vi "VI Properties Editor.vi"() -> ()   [LabVIEW 2020, in "VI Properties Editor.lvlib"]
doc: "Displays a window to add and edit properties and documentation of VIs and their individual controls."
uses:
  VI Properties Editor.lvlib
  Classes/Tree Map/Project Tree Map.lvclass
  Classes/Item/Item.lvclass
  CTLs/Main State Data.ctl
  CTLs/Main Front Panel Controls.ctl
  CTLs/Config.ctl
  <vilib>/Utility/miscctls.llb/LVSelectionTypeDef.ctl
  CTLs/Filter Type.ctl
  CTLs/Filter Column.ctl
  CTLs/Filter Info.ctl
  CTLs/Main References.ctl
  CTLs/Sort Info.ctl
  CTLs/Sort Column.ctl
panel:
  in  "Source Tree":string(tree)
  in  "Help Used":enum32{"Local Help File", "Web-based Help"}(tab)
  in  "Help tag":string
  in  "Help path":string
  in  "Help URL":string
  in  "View Saved Value":bool
  out "VI Type":string
  in  "Edit Icon":bool
  out "Preferred Exec System":string
  out "Priority":string
  out "Suspend when called?":bool
  out "Run when opened?":bool
  out "Auto error handling?":bool
  out "Allow debugging?":bool
  out "Reentrancy":string
  in  "Same as VI name":bool
  in  "Window title":string
  in  "Add Copyright":bool
  out "Inlined?":bool
  in  "Set all VIs":bool
  out "Location":string
  in  "VI description":string
  out "VI Connector Pane":picture
  in  "Controls":string[][](table)
  out "Current Filter":string
  out "Current Counts":string
  out "Current Source":string
  # "Select a VI to view/edit properties:"
  # "Controls"
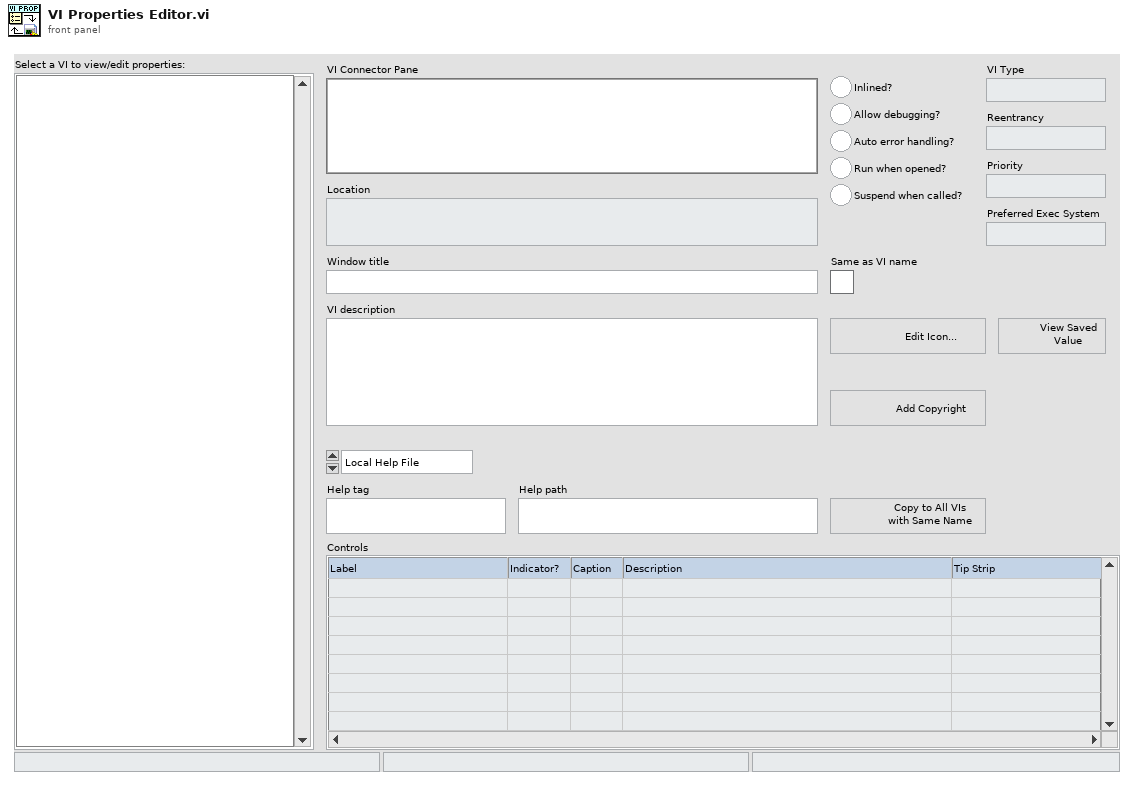
[diagram p1: front panel]
types:
  T1 = typedef "VI Properties Editor.lvlib/Main State Data.ctl" = cluster{"Core":cluster{"Current VI Reference":refnum<vi>, "Close Panel on Exit?":bool}, "FP Refs":T2, "Current Path":path, "New Item Data":refnum<class "Item.lvclass">[], "Saved Item Data":refnum<class "Item.lvclass">[], "FP":T3, "Config Path":path, "Config":T4, "Desc Selection":T8, "Displayed Indices":i32[], "Filter":T5, "Sort":T9, "Tree Map":refnum<class "Project Tree Map.lvclass">, "Last Save Count":u32, "View Saved?":bool, "Selected Item":refnum<class "Item.lvclass">}
  T2 = typedef "VI Properties Editor.lvlib/Main References.ctl" = cluster{"VI Tree":refnum<vi>, "Window Title":refnum<vi>, "Same Title as VI?":refnum<vi>, "VI Desc":refnum<vi>, "Help Path":refnum<vi>, "Help Tag":refnum<vi>, "Help URL":refnum<vi>, "Controls":refnum<vi>, "VI Connector Pane":refnum<vi>, "Path to VI":refnum<vi>, "Inlined?":refnum<vi>, "Allow Debugging?":refnum<vi>, "Auto Error Handling?":refnum<vi>, "Run When Opened?":refnum<vi>, "Suspend When Called?":refnum<vi>, "Reentrancy":refnum<vi>, "Priority":refnum<vi>, "Preferred Exec System":refnum<vi>, "VI Type":refnum<vi>, "Edit Icon":refnum<vi>, "Add Copyright":refnum<vi>, "Set all VIs":refnum<vi>, "Help Used":refnum<vi>}
  T3 = typedef "VI Properties Editor.lvlib/Main Front Panel Controls.ctl" = cluster{"Selected VI Data":i32, "Help Path":string, "Help Tag":string, "Help URL":string, "Help Type":enum16{"Local Help File", "Web-based Help"}, "VI Desc":string, "Controls":string[][], "Window Title":string, "Same Title?":bool, "VI Tree Value":string}
  T4 = typedef "VI Properties Editor.lvlib/Config.ctl" = cluster{"ItemsEdited":u32, "Copyright Path":path, "Copyright Delimiter":string, "Recent Folders":path[], "Recent Files":path[], "Recent Filters":T5[], "Abbreviate Names?":bool, "Format Bold Tags?":bool, "Show ConPane Only?":bool, "Show Top-Level Only?":bool, "Confirm Save?":bool, "Confirm Revert?":bool, "Confirm Save All?":bool, "Confirm Revert All?":bool, "Confirm Exit?":bool, "Flat View?":bool, "Ctls Sort Column":i32, "Ctls Sort Order":i32}
  T5 = typedef "VI Properties Editor.lvlib/Filter Info.ctl" = cluster{"Filter Column":T6, "Filter Type":T7, "Filter Value":string, "New Data?":bool, "Case Sensitive?":bool, "Enabled?":bool}
  T6 = typedef "VI Properties Editor.lvlib/Filter Column.ctl" = enum16{"Name", "Path", "Type", "Window Title", "Description", "Help Path", "Help Tag", "Custom Title?", "Reentrancy", "Inlined?", "Help URL", "Help Type", "Allow Debugging?", "Auto Error Handling?", "Run When Opened?", "Suspend When Called?", "Priority", "Preferred Exec Sytem", "Control Label", "Control Caption", "Control Description", "Control Tip Strip"}
  T7 = typedef "VI Properties Editor.lvlib/Filter Type.ctl" = enum16{"Contains", "Equals", "Starts with", "Ends with", "Is empty", "Does not contain", "Does not equal", "Is not empty"}
  T8 = typedef "LVSelectionTypeDef.ctl" = cluster{"Selection Start":u32, "Selection End":u32}
  T9 = typedef "VI Properties Editor.lvlib/Sort Info.ctl" = cluster{"Sort Column":T10, "Ascending?":bool, "Enabled?":bool}
  T10 = typedef "VI Properties Editor.lvlib/Sort Column.ctl" = enum16{"Name", "Filename", "Path", "Type", "Window Title", "Description", "Help Path", "Help Tag", "Custom Title?", "Reentrancy", "Inlined?", "Help URL", "Help Type", "Allow Debugging?", "Auto Error Handling?", "Run When Opened?", "Suspend When Called?", "Priority", "Preferred Exec Sytem"}
  T11 = enum16{"Text", "Background", "Item Symbol", "Open/Close Symbol", "Hierarchy Lines", "Right Border", "Bottom Border", "Bottom Right Corner", "Unknown Part"}
  T12 = typedef "LVPoint32TypeDef.ctl" = cluster{"Horizontal":i32, "Vertical":i32}
  T13 = cluster{"State(s) at Back":string, "Variant":variant}
  T14 = enum32{"Invalid", "Standard", "Closed", "Hidden", "Minimized", "Maximized"}
  T15 = enum32{"invalid app kind", "Development System", "Run Time System", "Student Edition", "Embedded LabVIEW", "Evaluation", "Custom"}
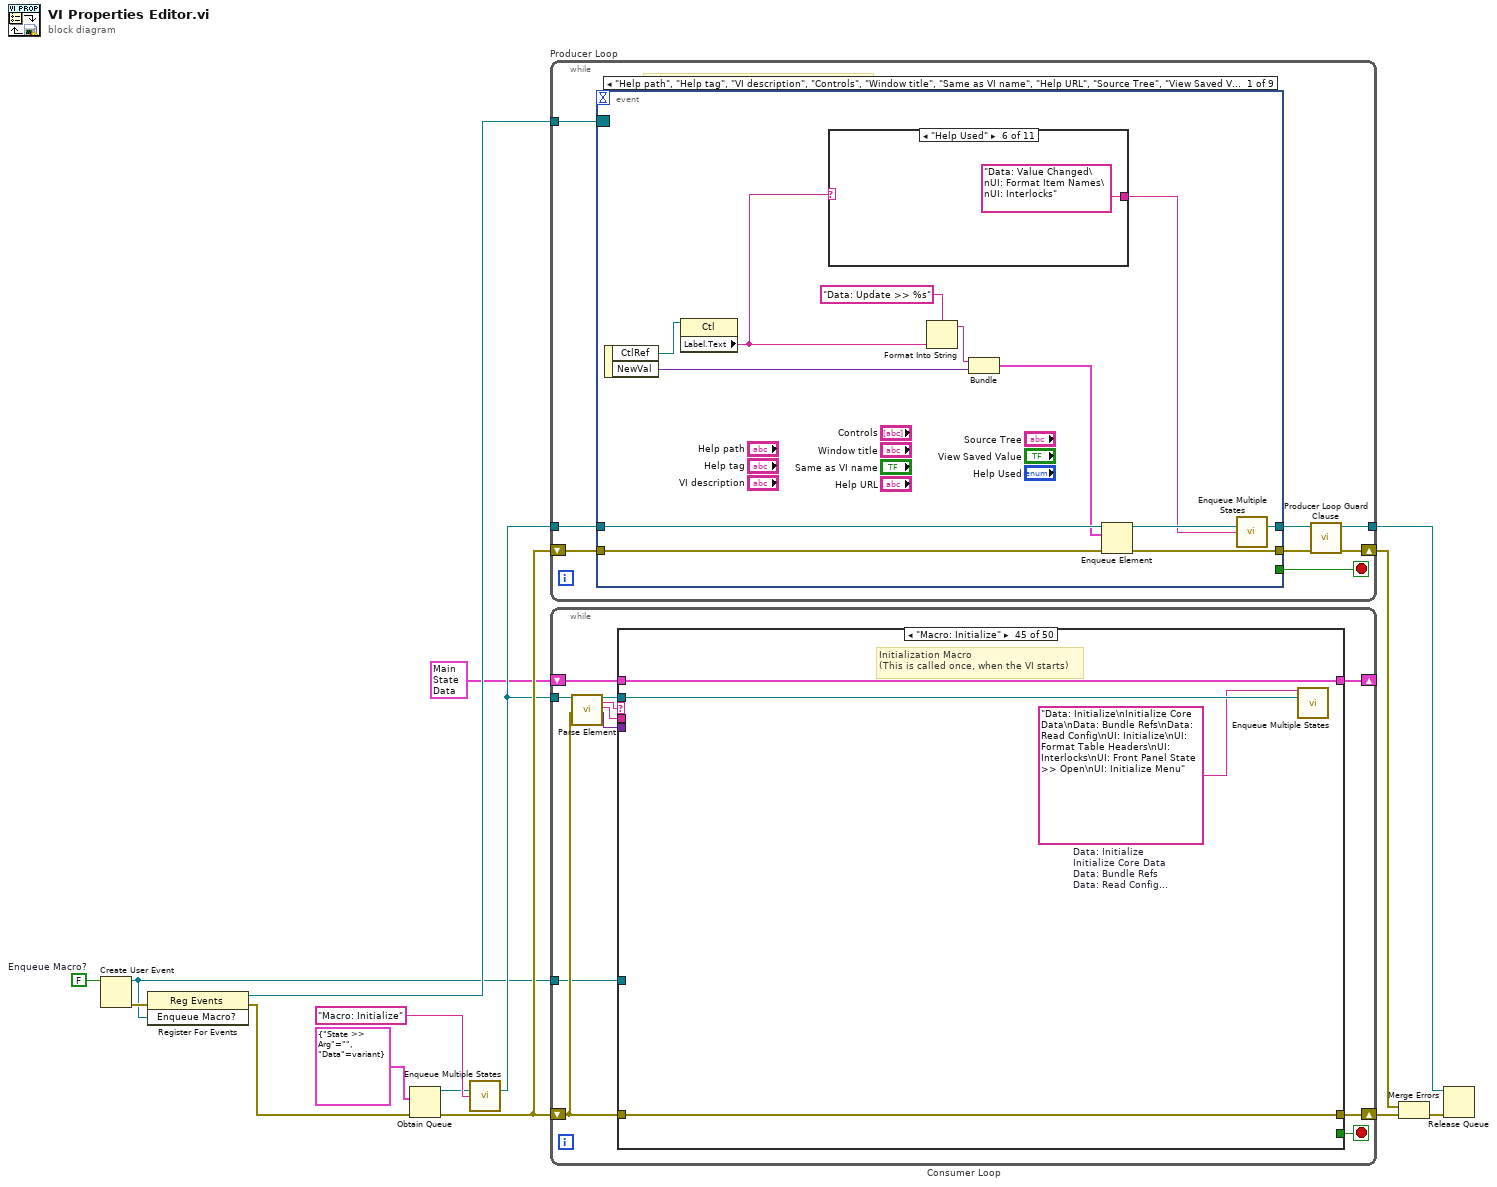
[diagram p0: block diagram]
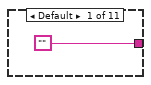
[diagram p2: hidden frame]
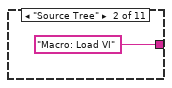
[diagram p3: hidden frame]
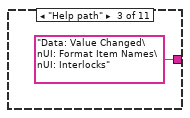
[diagram p4: hidden frame]
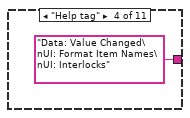
[diagram p5: hidden frame]
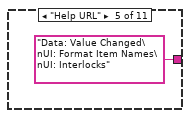
[diagram p6: hidden frame]
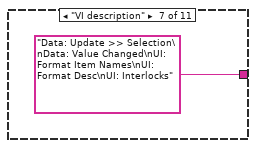
[diagram p7: hidden frame]
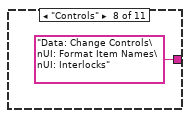
[diagram p8: hidden frame]
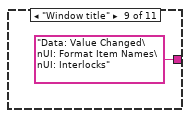
[diagram p9: hidden frame]
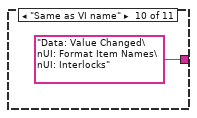
[diagram p10: hidden frame]
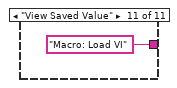
[diagram p11: hidden frame]
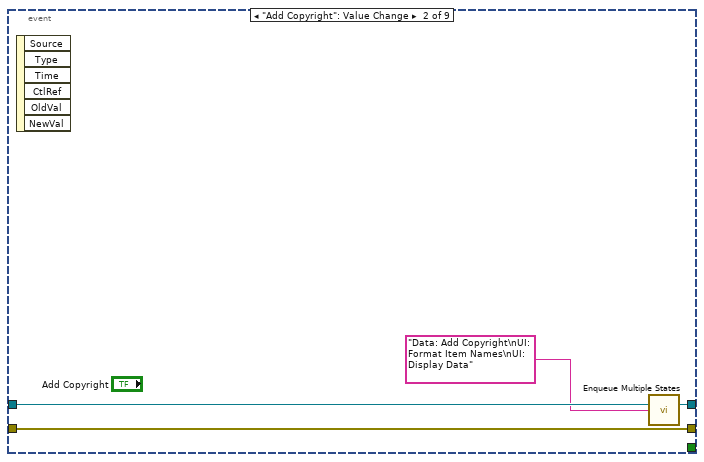
[diagram p12: hidden frame]
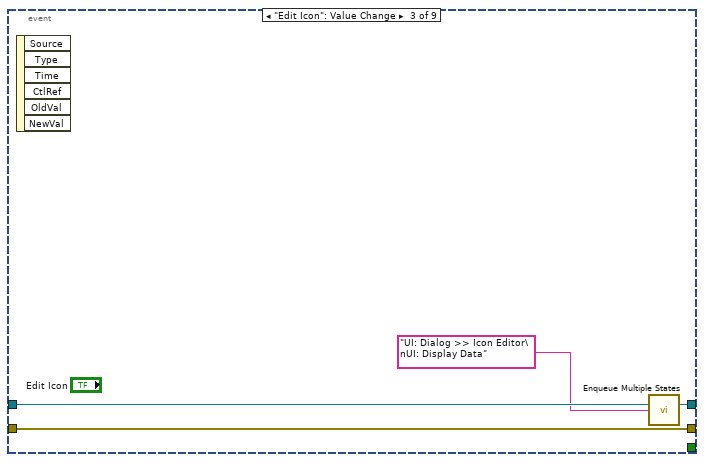
[diagram p13: hidden frame]
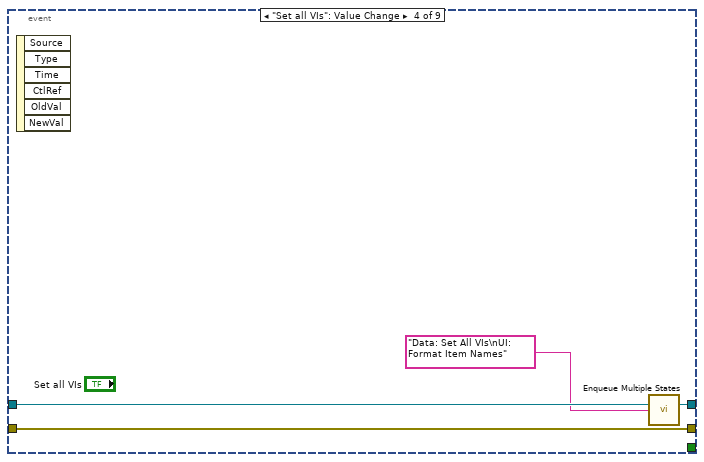
[diagram p14: hidden frame]
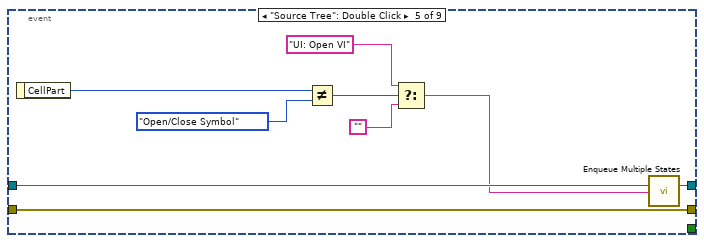
[diagram p15: hidden frame]
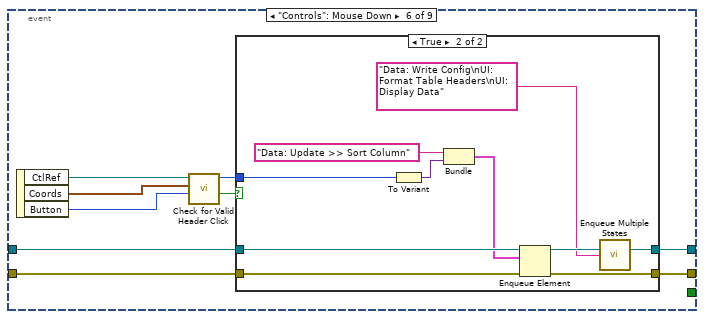
[diagram p16: hidden frame]
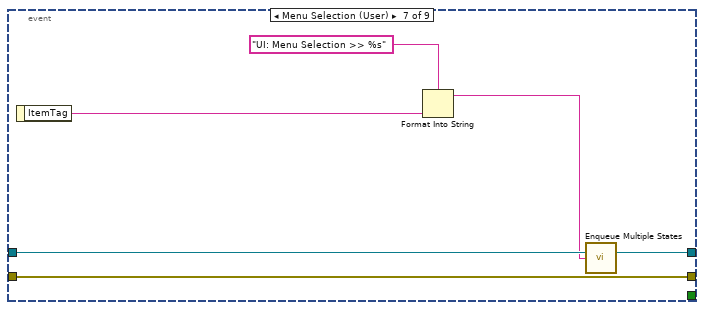
[diagram p18: hidden frame]
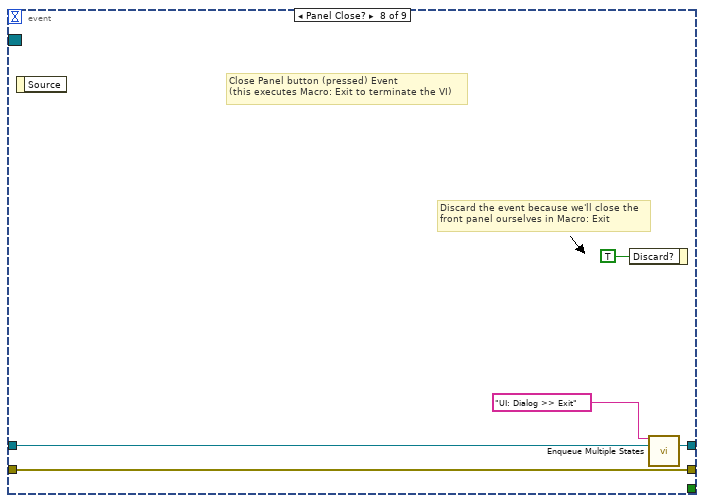
[diagram p19: hidden frame]
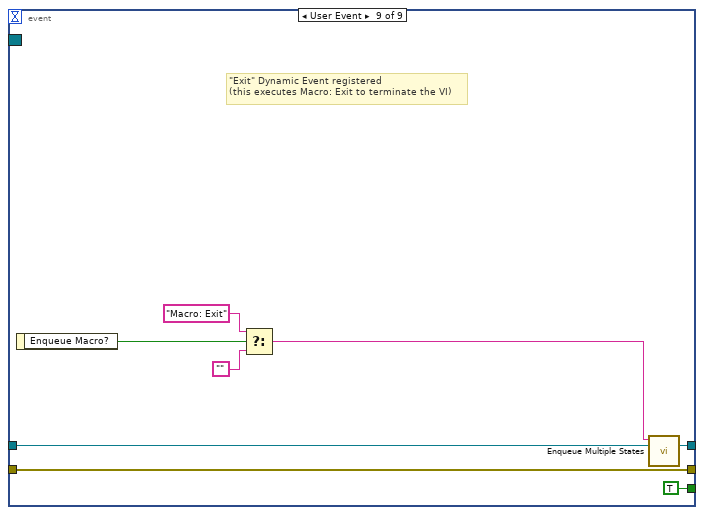
[diagram p20: hidden frame]
diagram:
  w5 = FALSE  # Enqueue Macro?
  n1 = Create User Event(user event datatype=w5) -> (user event=w2:refnum<user-event>, error out=w6:errorcluster)  [unwired: 1 in]
  n2 = register-events(error in=w6, w2) -> (reference out=w3:refnum<event-registration>, error out=w4:errorcluster)  [unwired: 1 in]
  n3 = Obtain Queue(element data type=cluster{"State >> Arg":string, "Data":variant} {"State >> Arg"="", "Data"=variant}, error in (no error)=w4) -> (queue out=w12:refnum<queue>, error out=w15:errorcluster)  [unwired: 3 in, 1 out]
  n4 = call "Enqueue Multiple States.vi"("queue in"=w12, "State(s) at Back"="Macro: Initialize") -> ("queue out"=w11:refnum<queue>)  [unwired: 13 in]
  n5 = while "Producer Loop" {
    shift-right: [w19] -> w9
    shift-left: w15 -> [w23]
    tunnel: w3 -> [w16]
    tunnel: w11 -> [w22]
    tunnel: [w17] -> w7
    stop <- w21 stop-if-true
    # "executes when the state queue is empty"
    n6 = event shown="[0] \"Help path\", \"Help tag\", \"VI description\", \"Controls\", \"Window title\", \"Same as VI name\", \"Help URL\", \"Source Tree\", \"View Saved Value\", \"Help Used\": Value Change" {
      selector: w16 -> [_ _ _ _ _ _ _ _ _]
      dyn-events: _ -> [_ _ _ _ _ _ _ _ _]
      timeout: _ -> [_ _ _ _ _ _ _ _ _]
      tunnel: [w33 w48 w52 w56 w65 w75 w92 w99 w107] -> w20
      tunnel: w23 -> [w34 w48 w52 w56 w65 w76 w92 w99 w107]
      tunnel: w22 -> [w32 w49 w53 w57 w66 w74 w91 w96 w106]
      tunnel: [w35 w50 w54 w58 w67 w73 w90 w95 w105] -> w18
      tunnel: [_ _ _ _ _ _ _ _ TRUE] -> w21
      event "Help path", "Help tag", "VI description", "Controls", "Window title", "Same as VI name", "Help URL", "Source Tree", "View Saved Value", "Help Used": Value Change {
        n7 = event-data() -> ("CtlRef"=w30:refnum<vi>, "NewVal"=w24:variant)  [unwired: 1 in]
        n8 = property on="Property Node" class="Ctl"(reference=w30) -> ("Label.Text"=w26:string)  [unwired: 1 in, 2 out]
        n9 = case shown="\"Help Used\"" w26 {
          tunnel: ["" ("Empty String Constant") "Macro: Load VI" "Data: Value Changed\nUI: Format Item Names\nUI: Interlocks" "Data: Value Changed\nUI: Format Item Names\nUI: Interlocks" "Data: Value Changed\nUI: Format Item Names\nUI: Interlocks" "Data: Value Changed\nUI: Format Item Names\nUI: Interlocks" "Data: Update >> Selection\nData: Value Changed\nUI: Format Item Names\nUI: Format Desc\nUI: Interlocks" "Data: Change Controls\nUI: Format Item Names\nUI: Interlocks" "Data: Value Changed\nUI: Format Item Names\nUI: Interlocks" "Data: Value Changed\nUI: Format Item Names\nUI: Interlocks" "Macro: Load VI"] -> w25
          frame Default {
          }
          frame "Source Tree" {
          }
          frame "Help path" {
          }
          frame "Help tag" {
          }
          frame "Help URL" {
          }
          frame "Help Used" {
          }
          frame "VI description" {
          }
          frame "Controls" {
          }
          frame "Window title" {
          }
          frame "Same as VI name" {
          }
          frame "View Saved Value" {
          }
        }
        n10 = Format Into String(format string="Data: Update >> %s", w26) -> (resulting string=w28:string)  [unwired: 2 in, 1 out]
        n11 = Bundle(w28, "NewVal"=w24) -> (w27:cluster{string, "NewVal":variant})  [unwired: 1 in]
        n12 = Enqueue Element(queue=w32, element=w27, error in (no error)=w34) -> (queue out=w31:refnum<queue>, error out=w33:errorcluster)  [unwired: 1 in, 1 out]
        n13 = call "Enqueue Multiple States.vi"("queue in"=w31, "State(s) at Back"=w25) -> ("queue out"=w35:refnum<queue>)  [unwired: 13 in]
      }
      event "Add Copyright": Value Change {
        n14 = event-data() -> ()  [unwired: 1 in, 6 out]
        n15 = call "Enqueue Multiple States.vi"("queue in"=w49, "State(s) at Back"="Data: Add Copyright\nUI: Format Item Names\nUI: Display Data") -> ("queue out"=w50:refnum<queue>)  [unwired: 13 in]
      }
      event "Edit Icon": Value Change {
        n16 = event-data() -> ()  [unwired: 1 in, 6 out]
        n17 = call "Enqueue Multiple States.vi"("queue in"=w53, "State(s) at Back"="UI: Dialog >> Icon Editor\nUI: Display Data") -> ("queue out"=w54:refnum<queue>)  [unwired: 13 in]
      }
      event "Set all VIs": Value Change {
        n18 = event-data() -> ()  [unwired: 1 in, 6 out]
        n19 = call "Enqueue Multiple States.vi"("queue in"=w57, "State(s) at Back"="Data: Set All VIs\nUI: Format Item Names") -> ("queue out"=w58:refnum<queue>)  [unwired: 13 in]
      }
      event "Source Tree": Double Click {
        n20 = event-data() -> ("CellPart"=w64:T11)  [unwired: 1 in]
        n21 = Not Equal?(x=w64, y=T11."Open/Close Symbol") -> (x != y?=w62:bool)
        n22 = Select(t="UI: Open VI" ("State(s) at Back"), s=w62, f="" ("Empty String Constant")) -> (s? t:f=w59:string)
        n23 = call "Enqueue Multiple States.vi"("queue in"=w66, "State(s) at Back"=w59) -> ("queue out"=w67:refnum<queue>)  [unwired: 13 in]
      }
      event "Controls": Mouse Down {
        n24 = event-data() -> ("CtlRef"=w72:refnum<vi>, "Coords"=w71:T12, "Button"=w70:u16)  [unwired: 1 in]
        n25 = call "Check for Valid Header Click.vi"("Button"=w70, "Coords"=w71, "Table Ref"=w72) -> ("Valid Click?"=w69:bool, "Column"=w68:i32)  [unwired: 7 in]
        n26 = case shown="True" w69 {
          tunnel: w76 -> [w77 w88]
          tunnel: [w77 w87] -> w75
          tunnel: w74 -> [w78 w85]
          tunnel: [w78 w84] -> w73
          tunnel: w68 -> [_ w81]
          frame False {
          }
          frame True {
            n27 = To Variant(anything=w81) -> (Variant=w83:variant)
            n28 = Bundle("State(s) at Back"="Data: Update >> Sort Column", "Variant"=w83) -> (w80:T13)  [unwired: 1 in]
            n29 = Enqueue Element(queue=w85, element=w80, error in (no error)=w88) -> (queue out=w86:refnum<queue>, error out=w87:errorcluster)  [unwired: 1 in, 1 out]
            n30 = call "Enqueue Multiple States.vi"("queue in"=w86, "State(s) at Back"="Data: Write Config\nUI: Format Table Headers\nUI: Display Data") -> ("queue out"=w84:refnum<queue>)  [unwired: 13 in]
          }
        }
      }
      event Menu Selection (User) {
        n31 = event-data() -> ("ItemTag"=w93:string)  [unwired: 1 in]
        n32 = Format Into String(format string="UI: Menu Selection >> %s", w93) -> (resulting string=w89:string)  [unwired: 2 in, 1 out]
        n33 = call "Enqueue Multiple States.vi"("queue in"=w91, "State(s) at Back"=w89) -> ("queue out"=w90:refnum<queue>)  [unwired: 13 in]
      }
      event Panel Close? {
        # "Discard the event because we'll close the front panel ourselves in Macro: Exit"
        # "Close Panel button (pressed) Event\n(this executes Macro: Exit to terminate the VI)"
        n34 = event-data() -> ()  [unwired: 1 in, 1 out]
        n35 = event-data ("Event Filter Node")("Discard?"=TRUE) -> ()  [unwired: 1 in, 1 out]
        n36 = call "Enqueue Multiple States.vi"("State(s) at Front"="UI: Dialog >> Exit", "queue in"=w96) -> ("queue out"=w95:refnum<queue>)  [unwired: 13 in]
      }
      event User Event {
        # "\"Exit\" Dynamic Event registered\n(this executes Macro: Exit to terminate the VI)"
        n37 = event-data() -> ("Enqueue Macro?"=w103:bool)  [unwired: 1 in]
        n38 = Select(t="Macro: Exit", s=w103, f="" ("Empty String Constant")) -> (s? t:f=w100:string)
        n39 = call "Enqueue Multiple States.vi"("State(s) at Front"=w100, "queue in"=w106) -> ("queue out"=w105:refnum<queue>)  [unwired: 13 in]
      }
    }
    n40 = call "Producer Loop Guard Clause.vi"("error in (no error)"=w20, "queue in"=w18) -> ("error out"=w19:errorcluster, "queue out"=w17:refnum<queue>)  [unwired: 8 in]
  }
  n41 = while "Consumer Loop" {
    shift-right: [w115] -> _
    shift-left: T1 {"Core"={"Current VI Reference"=refnum, "Close Panel on Exit?"=FALSE}, "FP Refs"={"VI Tree"=refnum, "Window Title"=refnum, "Same Title as VI?"=refnum, "VI Desc"=refnum, "Help Path"=refnum, "Help Tag"=refnum, "Help URL"=refnum, "Controls"=refnum, "VI Connector Pane"=refnum, "Path to VI"=refnum, "Inlined?"=refnum, "Allow Debugging?"=refnum, "Auto Error Handling?"=refnum, "Run When Opened?"=refnum, "Suspend When Called?"=refnum, "Reentrancy"=refnum, "Priority"=refnum, "Preferred Exec System"=refnum, "VI Type"=refnum, "Edit Icon"=refnum, "Add Copyright"=refnum, "Set all VIs"=refnum, "Help Used"=refnum}, "Current Path"=path "", "New Item Data"=[], "Saved Item Data"=[], "FP"={"Selected VI Data"=0, "Help Path"="", "Help Tag"="", "Help URL"="", "Help Type"=enum."Local Help File", "VI Desc"="", "Controls"=[], "Window Title"="", "Same Title?"=FALSE, "VI Tree Value"=""}, "Config Path"=path "", "Config"={"ItemsEdited"=0, "Copyright Path"=path "", "Copyright Delimiter"="", "Recent Folders"=[], "Recent Files"=[], "Recent Filters"=[], "Abbreviate Names?"=FALSE, "Format Bold Tags?"=FALSE, "Show ConPane Only?"=FALSE, "Show Top-Level Only?"=FALSE, "Confirm Save?"=FALSE, "Confirm Revert?"=FALSE, "Confirm Save All?"=FALSE, "Confirm Revert All?"=FALSE, "Confirm Exit?"=FALSE, "Flat View?"=FALSE, "Ctls Sort Column"=0, "Ctls Sort Order"=0}, "Desc Selection"={"Selection Start"=0, "Selection End"=0}, "Displayed Indices"=[], "Filter"={"Filter Column"=enum."Name", "Filter Type"=enum."Contains", "Filter Value"="", "New Data?"=FALSE, "Case Sensitive?"=FALSE, "Enabled?"=FALSE}, "Sort"={"Sort Column"=enum."Name", "Ascending?"=FALSE, "Enabled?"=FALSE}, "Tree Map"=refnum, "Last Save Count"=0, "View Saved?"=FALSE, "Selected Item"=refnum} ("VI Properties Editor State Data") -> [w114]
    shift-right: [w118] -> w10
    shift-left: w15 -> [w117]
    tunnel: w11 -> [w113]
    tunnel: w2 -> [w108]
    stop <- w116 stop-if-true
    n42 = call "Parse Element.vi"("queue in"=w113, "error in (no error)"=w117) -> ("queue out"=w112:refnum<queue>, "State"=w111:string, "Arg"=w110:string, "Data"=w109:variant)  [unwired: 14 in]
    n43 = case shown="\"Macro: Initialize\"" w111 {
      selector: w111 -> [_ w121 _ _ _ _ _ _ _ _ _ _ _ _ _ _ _ _ _ _ _ _ _ _ _ _ _ _ _ _ _ _ _ _ _ _ _ _ _ _ _ _ _ _ _ _ _ _ _ _]
      tunnel: w112 -> [_ _ _ _ _ _ _ _ _ w216 _ w223 _ _ _ _ _ _ _ _ _ _ _ _ _ _ _ w399 _ _ _ _ w502 _ _ w544 _ _ _ _ _ _ _ _ w662 w666 w671 w684 w691 w703]
      tunnel: w110 -> [_ _ _ w146 _ _ _ _ w201 _ _ w224 w232 _ _ _ _ _ _ _ _ w353 _ _ _ _ _ w394 w401 w409 w481 _ w497 _ _ w531 _ _ _ _ _ w612 w651 _ _ _ w670 w682 w689 _]
      tunnel: w114 -> [w119 w123 w140 w150 w153 w155 w169 w199 w203 w212 w219 w227 w235 w262 w277 w286 w294 w300 w311 w332 w340 w356 w370 w374 w377 w388 w390 w400 w402 w411 w486 w494 w499 w523 w529 w542 w560 w573 w584 w595 w603 w610 w649 w659 w663 w667 w672 w681 w688 w707]
      tunnel: [w120 w128 w145 errorcluster {"status"=FALSE, "code"=0, "source"=""} ("error out") w154 w156 w162 w197 w204 w214 w220 w228 w238 w259 w278 w287 w295 w298 w308 w333 w341 w362 w372 w375 w378 w380 w392 w397 w403 w412 w482 w491 w500 w518 w527 w533 w561 w574 w580 w591 w602 w615 w653 w660 w664 w668 w673 w680 w687 w696] -> w118
      tunnel: w117 -> [w120 w127 w145 w149 w154 w156 w161 w197 w205 w215 w221 w229 w237 w260 w278 w287 w295 w299 w309 w333 w341 w358 w373 w375 w378 w383 w393 w398 w404 w413 w483 w492 w501 w514 w528 w535 w562 w575 w581 w592 w607 w614 w652 w660 w664 w668 w673 w680 w687 w708]
      tunnel: [_ _ _ _ TRUE _ _ _ _ _ _ _ _ _ _ _ _ _ _ _ _ _ _ _ _ _ _ _ _ _ _ _ _ _ _ _ _ _ _ _ _ _ _ _ _ _ _ _ _ _] -> w116
      tunnel: [w119 w123 w144 w150 w153 w155 w168 w198 w202 w213 w219 w227 w234 w261 w276 w285 w293 w297 w312 w334 w342 w361 w370 w374 w377 w388 w390 w400 w402 w411 w486 w494 w498 w523 w529 w541 w560 w573 w583 w594 w603 w611 w650 w659 w663 w667 w672 w681 w688 w707] -> w115
      tunnel: w109 -> [_ _ _ w147 _ _ _ _ w200 _ _ _ _ _ _ _ _ _ _ _ _ _ _ _ _ _ _ _ _ _ _ _ _ _ _ _ _ _ _ _ _ _ _ _ _ _ _ _ _ _]
      tunnel: w108 -> [_ _ _ _ _ _ _ _ _ _ _ _ _ _ _ _ _ _ _ _ _ _ _ _ _ _ _ _ _ _ _ _ _ _ _ _ _ _ _ _ _ _ _ _ _ _ _ _ _ w699]
      frame "---------- Core ----------" {
        # "Do not put any code in this frame.\n(it is a separator no-op)"
      }
      frame Default {
        w125 = 42 items=["No error", "Argument error", "Memory is full", "Out of zone", "End of file", "File already open", "Generic file I/O error", "File not found", "File permission error", "Disk is full", "Duplicate path", "Too many files open", "System feature not enabled", "Resource file not found", "Cannot add resource", "Resource not found", "Image not found", "Image memory error", "Pen does not exist", "Config type invalid", "Config token not found", "Config parse error", "Config memory error", "Bad external code format", "Bad external code offset", "External code not present", "Null window", "Destroy window error", "Null menu", "Print aborted", "Bad print record", "Print driver error", "Windows error during printing", "Memory error during printing", "Print dialog error", "Generic print error", "Invalid device refnum", "Device not found", "Device parameter error", "Device unit error", "Cannot open device", "Device call aborted", "Generic error", "Cancelled by user", "Object ID too low", "Object ID too high", "Object not in heap", "Unknown heap", "Unknown object (invalid DefProc)", "Unknown object (DefProc not in table)", "Message out of range", "Invalid (null) method", "Unknown message", "Manager call not supported", "Bad address", "Network operation in progress", "Network operation timed out", "Connection is busy", "Network attribute not supported", "Network error", "Address in use", "System out of memory", "Connection aborted", "Connection refused", "Not connected", "Already connected", "Connection closed", "Initialization error (interapplication manager)", "Bad occurrence", "Wait on unbound occurrence handler", "Occurrence queue overflow", "Datalog type conflict", "Unused", "Unrecognized type (interapplication manager)", "Memory corrupt", "Failed to make temporary DLL", "Old CIN version", "Drag socket not found", "Failed to load drop-object", "Failed to register OLE object", "Failed to release OLE object", "Format specifier type mismatch", "Unknown format specifier", "Too few format specifiers", "Too many format specifiers", "Scan failed", "Newer CIN version", "Error converting to variant", "Runtime menu error", "Password tampered", "Variant attribute not found", "Incompatible variant data type", "Event data is not available", "Event Store is not present", "Occurrence is not found", "Event Queue is not created", "Event info is not available", "Refnum passed is NULL", "Error retrieving Class GUID", "Error retrieving CoClass GUID", "Error retrieving TypeLib GUID.", "Bad built application magic bytes.", "Specific driver is different from the specific driver associated with the Logical Name.", "There is no session opened to the class driver.", "Max Error", "MAX - Error with config objects", "MAX - Error loading configuration", "MAX - Group not supported"]
        # "Current State"
        # "Do not delete, rename, or modify this frame.\n(this is used to capture unhandled states and typos)"
        # "Handle mistyped state name (developer tool)"
        n44 = Format Into String(format string="Software Exception: Unhandled State \"%s\"." ("message"), error in=w127, w121) -> (resulting string=w124:string, error out=w129:errorcluster)  [unwired: 1 in]
        n45 = call <vilib>:"Error Cluster From Error Code.vi"("show call chain? (False)"=TRUE, "error in (no error)"=w129, "error message (\"\")"=w124, "error code (0)"=w125) -> ("error out"=w128:errorcluster)  [unwired: 5 in]
      }
      frame "Initialize Core Data" {
        # "Want the VI to close when ran from the Tools menu"
        # "originally closed?"
        # "exe?"
        # "If panel starts closed or is an EXE, then close it when we exit"
        n46 = property on="Property Node" class="VI"() -> ("FP.State"=w137:T14)  [unwired: 2 in, 2 out]
        n47 = property on="Property Node" class="App"() -> ("App.Kind"=w143:T15)  [unwired: 2 in, 2 out]
        n48 = Current VI's Path() -> (path=w134:path)
        n49 = control-ref of="Current VI Reference"() -> (w138:refnum<vi>)
        n50 = Strip Path(path=w134) -> (stripped path=w133:path)  [unwired: 1 out]
        n51 = Equal?(x=w137, y=T14."Closed" ("Front Panel Window:State")) -> (x = y?=w135:bool)
        n52 = Equal?(x=w143, y=T15."Run Time System" ("Application:Kind")) -> (x = y?=w141:bool)
        n53 = Strip Path(path=w133) -> (name=w132:string)  [unwired: 1 out]
        n54 = Equal?(x=w132, y="Redhawk" ("name")) -> (x = y?=w130:bool)
        n55 = Compound Arithmetic op=OR(w135, w141, w130) -> (w139:bool)
        n56 = Bundle By Name(cluster=w140, "Core.Current VI Reference"=w138, "Core.Close Panel on Exit?"=w139) -> (w144:T1)
      }
      frame "Error Handler" {
        # "Unhandled Error -- Display it"
        # "Handle any errors here.\nYou can also output any states to clean-up after errors occur"
        # "Clear error"
        n57 = call "Build Error Message.vi"("error in (no error)"=w149, "Data"=w147, "Arg"=w146) -> ("error out"=w148:errorcluster)  [unwired: 8 in]
        n58 = call <vilib>:"General Error Handler.vi"("error in (no error)"=w148) -> ()  [unwired: 10 in, 5 out]
      }
      frame "Exit" {
        # "Do not put any code in this frame.\n(No errors that occur here will be handled.)"
      }
      frame "---------- Data ----------" {
        # "Do not put any code in this frame.\n(It is a separator no-op. You can make a copy of this frame to create a new Data frame)"
      }
      frame "Data: Initialize" {
        # "Initialize the shift-register data, here."
        n59 = call "Config Path--constant.vi"() -> ("Config Path"=w158:path)  [unwired: 11 in]
        n60 = Strip Path(path=w158) -> (stripped path=w166:path)  [unwired: 1 out]
        n61 = call <vilib>:"Check if File or Folder Exists.vi"("error in (no error)"=w161, "path"=w166) -> ("error out"=w165:errorcluster, "file or folder exists?"=w163:bool, "dup path"=w164:path)  [unwired: 7 in]
        n62 = case shown="True" w163 {
          tunnel: [w172 w173] -> w162
          tunnel: w165 -> [w171 w173]
          tunnel: w164 -> [w170 _]
          frame False {
            n63 = Create Folder(path (use dialog)=w170, error in=w171) -> (error out=w172:errorcluster)  [unwired: 1 in, 2 out]
          }
          frame True {
          }
        }
        n64 = Bundle By Name(cluster=w169, "FP.Selected VI Data"=-1 ("FP.VI Selected"), "Sort.Sort Column"=Sort_Column."Name", "Sort.Ascending?"=TRUE ("Ascending?"), "Sort.Enabled?"=FALSE ("Ascending?"), "Config Path"=w158) -> (w168:T1)
      }
      frame "Data: Bundle Refs" {
        n65 = control-ref of="Source Tree"() -> (w196:refnum<vi>)
        n66 = control-ref of="Help Used"() -> (w178:refnum<vi>)
        n67 = control-ref of="Same as VI name"() -> (w194:refnum<vi>)
        n68 = control-ref of="Inlined?"() -> (w186:refnum<vi>)
        n69 = control-ref of="Allow debugging?"() -> (w185:refnum<vi>)
        n70 = control-ref of="Auto error handling?"() -> (w184:refnum<vi>)
        n71 = control-ref of="Run when opened?"() -> (w183:refnum<vi>)
        n72 = control-ref of="Suspend when called?"() -> (w182:refnum<vi>)
        n73 = control-ref of="Edit Icon"() -> (w177:refnum<vi>)
        n74 = control-ref of="Add Copyright"() -> (w176:refnum<vi>)
        n75 = control-ref of="Set all VIs"() -> (w175:refnum<vi>)
        n76 = control-ref of="VI Connector Pane"() -> (w189:refnum<vi>)
        n77 = control-ref of="Window title"() -> (w195:refnum<vi>)
        n78 = control-ref of="VI description"() -> (w193:refnum<vi>)
        n79 = control-ref of="Help path"() -> (w192:refnum<vi>)
        n80 = control-ref of="Help tag"() -> (w191:refnum<vi>)
        n81 = control-ref of="Help URL"() -> (w187:refnum<vi>)
        n82 = control-ref of="Location"() -> (w188:refnum<vi>)
        n83 = control-ref of="Reentrancy"() -> (w181:refnum<vi>)
        n84 = control-ref of="Priority"() -> (w180:refnum<vi>)
        n85 = control-ref of="Preferred Exec System"() -> (w179:refnum<vi>)
        n86 = control-ref of="VI Type"() -> (w174:refnum<vi>)
        n87 = control-ref of="Controls"() -> (w190:refnum<vi>)
        n88 = Bundle By Name(cluster=w199, "FP Refs.VI Tree"=w196, "FP Refs.Window Title"=w195, "FP Refs.Same Title as VI?"=w194, "FP Refs.VI Desc"=w193, "FP Refs.Help Path"=w192, "FP Refs.Help Tag"=w191, "FP Refs.Help URL"=w187, "FP Refs.Controls"=w190, "FP Refs.VI Connector Pane"=w189, "FP Refs.Path to VI"=w188, "FP Refs.Inlined?"=w186, "FP Refs.Allow Debugging?"=w185, "FP Refs.Auto Error Handling?"=w184, "FP Refs.Run When Opened?"=w183, "FP Refs.Suspend When Called?"=w182, "FP Refs.Reentrancy"=w181, "FP Refs.Priority"=w180, "FP Refs.Preferred Exec System"=w179, "FP Refs.VI Type"=w174, "FP Refs.Help Used"=w178, "FP Refs.Edit Icon"=w177, "FP Refs.Add Copyright"=w176, "FP Refs.Set all VIs"=w175) -> (w198:T1)
      }
      frame "Data: Update" {
        n89 = call "Update State Data.vi"("error in (no error)"=w205, "Data"=w200, "Argument"=w201, "State Data"=w203) -> ("error out"=w204:errorcluster, "State Data out"=w202:T1)  [unwired: 6 in]
      }
      frame "Data: Read Config" {
        n90 = Unbundle By Name(w212) -> ("Config Path"=w211:path)
        n91 = call "Read Config.vi"("error in (no error)"=w215, "Path"=w211) -> ("error out"=w214:errorcluster, "Config"=w210:T4, "File Created?"=w209:bool)  [unwired: 7 in]
        n92 = Bundle By Name(cluster=w212, "Config"=w210) -> (w213:T1)
        n93 = Select(t="Data: Write Config", s=w209, f="" ("Empty String Constant")) -> (s? t:f=w206:string)
        n94 = call "Enqueue Multiple States.vi"("queue in"=w216, "State(s) at Back"=w206) -> ()  [unwired: 13 in, 1 out]
      }
      frame "Data: Write Config" {
        n95 = Unbundle By Name(w219) -> ("Config Path"=w217:path, "Config"=w218:T4)
        n96 = call "Write Config.vi"("error in (no error)"=w221, "Config"=w218, "Path"=w217) -> ("error out"=w220:errorcluster)  [unwired: 8 in]
      }
      frame "Data: Check Source" {
        n97 = Unbundle By Name(w227) -> ("Config"=w226:T4, "Current Path"=w225:path)
        n98 = call "Check Data Source.vi"("error in (no error)"=w229, "Argument"=w224, "Current Path"=w225, "Config"=w226) -> ("error out"=w228:errorcluster, "States"=w222:string)  [unwired: 6 in]
        n99 = call "Enqueue Multiple States.vi"("queue in"=w223, "State(s) at Back"=w222) -> ()  [unwired: 13 in, 1 out]
      }
      frame "Data: Load VIs" {
        n100 = Unbundle By Name(w235) -> ("Core.Current VI Reference"=w230:refnum<vi>, "Current Path"=w236:path)
        n101 = Equal?(x=w232, y="Reload") -> (x = y?=w231:bool)
        n102 = in-place "In Place Element Structure" {
          in-place-border: [w249] -> w238
          in-place-border: w237 -> [w248]
          in-place-border: w236 -> [w242]
          in-place-border: w231 -> [w244]
          in-place-border: w230 -> [w243]
          n103 = in-place-cluster #1(w235) -> ("New Item Data"=w247:refnum<class "Item.lvclass">[], "Saved Item Data"=w240:refnum<class "Item.lvclass">[])
          n104 = call "Get All Items.vi"("Calling VI Ref"=w243, "error in (no error)"=w248, "Path"=w242) -> ("error out"=w249:errorcluster, "Cancelled?"=w241:bool, "Item Data"=w246:refnum<class "Item.lvclass">[])  [unwired: 6 in]
          n105 = case shown="False" w241 {
            tunnel: w247 -> [w256 w258]
            tunnel: w246 -> [w250 _]
            tunnel: [w255 w258] -> w245
            tunnel: w244 -> [w254 _]
            tunnel: w242 -> [w253 _]
            tunnel: w240 -> [_ w257]
            tunnel: [w250 w257] -> w239
            frame False {
              n106 = Array Size(array=w250) -> (size(s)=w252:i32)
              n107 = Select(t=w256, s=w254, f=w250) -> (s? t:f=w255:refnum<class "Item.lvclass">[])
              n108 = call "Format Current Source String.vi"("Item Count"=w252, "Current Path"=w253) -> ("Current Source String"=→"Current Source":string)  [unwired: 9 in]
            }
            frame True {
            }
          }
          n109 = in-place-cluster #1("New Item Data"=w245, "Saved Item Data"=w239) -> (w234:T1)
        }
      }
      frame "Data: Filter/Sort VIs" {
        n110 = in-place "In Place Element Structure" {
          in-place-border: w260 -> [w269]
          in-place-border: [w268] -> w259
          n111 = in-place-cluster #2(w262) -> ("Sort"=w273:T9, "Filter"=w274:T5, "Saved Item Data"=w265:refnum<class "Item.lvclass">[], "New Item Data"=w266:refnum<class "Item.lvclass">[])  [unwired: 1 out]
          n112 = call "Filter and Sort Items.vi"("Sort Info"=w273, "Filter Info"=w274, "error in (no error)"=w269, "New Item Data"=w266, "Saved Item Data"=w265) -> ("error out"=w268:errorcluster, "Displayed Indices"=w263:i32[], "New Item Data out"=w267:refnum<class "Item.lvclass">[], "Saved Item Data out"=w264:refnum<class "Item.lvclass">[])  [unwired: 3 in]
          n113 = call "Convert Filter to Display String.vi"("Filter Info"=w274) -> ("String"=w270:string)  [unwired: 10 in]
          n114 = Concatenate Strings("Current filter:  " ("string"), w270) -> (→"Current Filter":string)
          n115 = in-place-cluster #2("Sort"=w273, "Filter"=w274, "Saved Item Data"=w264, "New Item Data"=w267, "Displayed Indices"=w263) -> (w261:T1)
        }
      }
      frame "Data: Value Changed" {
        n116 = Unbundle By Name(w277) -> ("FP"=w275:T3)
        n117 = in-place "In Place Element Structure" {
          in-place-border: w275 -> [w280]
          n118 = in-place-cluster #3(w277) -> ("New Item Data"=w279:refnum<class "Item.lvclass">[])
          n119 = call "Set VI Properties.vi"("Front Panel Controls"=w280, "Item Data"=w279) -> ("Item Data out"=w281:refnum<class "Item.lvclass">[])  [unwired: 9 in]
          n120 = in-place-cluster #3("New Item Data"=w281) -> (w276:T1)
        }
      }
      frame "Data: Revert Current" {
        n121 = Unbundle By Name(w286) -> ("FP.Selected VI Data"=w282:i32, "Saved Item Data"=w284:refnum<class "Item.lvclass">[])
        n122 = Index Array(array=w284, index=w282) -> (element=w283:refnum<class "Item.lvclass">)
        n123 = in-place "In Place Element Structure" {
          in-place-border: w283 -> [w290]
          in-place-border: w282 -> [w289]
          n124 = in-place-cluster #4(w286) -> ("New Item Data"=w291:refnum<class "Item.lvclass">[])
          n125 = Replace Array Subset(array=w291, new element=w290, index=w289) -> (w288:refnum<class "Item.lvclass">[])
          n126 = in-place-cluster #4("New Item Data"=w288) -> (w285:T1)
        }
      }
      frame "Data: Revert All" {
        n127 = Unbundle By Name(w294) -> ("Saved Item Data"=w292:refnum<class "Item.lvclass">[])
        n128 = in-place "In Place Element Structure" {
          in-place-border: w292 -> [w296]
          n129 = in-place-cluster #5(w294) -> ()  [unwired: 1 out]
          n130 = in-place-cluster #5("New Item Data"=w296) -> (w293:T1)
        }
      }
      frame "Data: Save All" {
        n131 = in-place "In Place Element Structure" {
          in-place-border: w299 -> [w307]
          in-place-border: [w306] -> w298
          n132 = in-place-cluster #6(w300) -> ("New Item Data"=w303:refnum<class "Item.lvclass">[], "Saved Item Data"=w302:refnum<class "Item.lvclass">[])  [unwired: 1 out]
          n133 = call "Save All VI Data.vi"("error in (no error)"=w307, "Saved Item Data"=w302, "New Item Data"=w303) -> ("error out"=w306:errorcluster, "Items Saved"=w301:u32, "Saved Item Data out"=w304:refnum<class "Item.lvclass">[], "New Item Data out"=w305:refnum<class "Item.lvclass">[])  [unwired: 5 in]
          n134 = in-place-cluster #6("Last Save Count"=w301, "New Item Data"=w305, "Saved Item Data"=w304) -> (w297:T1)
        }
      }
      frame "Data: Save Current" {
        n135 = Unbundle By Name(w311) -> ("FP.Selected VI Data"=w310:i32)
        n136 = in-place "In Place Element Structure" {
          in-place-border: w310 -> [w318]
          in-place-border: w309 -> [w315]
          in-place-border: [w314] -> w308
          n137 = in-place-cluster #7(w311) -> ("New Item Data"=w320:refnum<class "Item.lvclass">[], "Saved Item Data"=w319:refnum<class "Item.lvclass">[])  [unwired: 1 out]
          n138 = in-place "In Place Element Structure" {
            in-place-border: w315 -> [w323]
            in-place-border: [w322] -> w314
            in-place-border: [w321] -> w313
            n139 = in-place-array #8(w320, w318) -> (w331:refnum<class "Item.lvclass">)
            n140 = in-place-array #9(w319, w318) -> (w330:refnum<class "Item.lvclass">)
            n141 = Build Array(w331) -> (w329:refnum<class "Item.lvclass">[])
            n142 = Build Array(w330) -> (w328:refnum<class "Item.lvclass">[])
            n143 = call "Save All VI Data.vi"("error in (no error)"=w323, "Saved Item Data"=w328, "New Item Data"=w329) -> ("error out"=w322:errorcluster, "Items Saved"=w321:u32, "Saved Item Data out"=w325:refnum<class "Item.lvclass">[], "New Item Data out"=w327:refnum<class "Item.lvclass">[])  [unwired: 5 in]
            n144 = Index Array(array=w327) -> (element=w326:refnum<class "Item.lvclass">)  [unwired: 1 in]
            n145 = Index Array(array=w325) -> (element=w324:refnum<class "Item.lvclass">)  [unwired: 1 in]
            n146 = in-place-array #8(w326) -> (w316:refnum<class "Item.lvclass">[])  [unwired: 1 out]
            n147 = in-place-array #9(w324) -> (w317:refnum<class "Item.lvclass">[])  [unwired: 1 out]
          }
          n148 = in-place-cluster #7("New Item Data"=w316, "Saved Item Data"=w317, "Last Save Count"=w313) -> (w312:T1)
        }
      }
      frame "Data: Set All VIs" {
        n149 = in-place "In Place Element Structure" {
          n150 = in-place-cluster #10(w332) -> ("FP"=w335:T3, "New Item Data"=w337:refnum<class "Item.lvclass">[])
          n151 = call "Copy to Matching Items.vi"("Front Panel Controls"=w335, "Item Data"=w337) -> ("Item Data out"=w336:refnum<class "Item.lvclass">[])  [unwired: 9 in]
          n152 = in-place-cluster #10("FP"=w335, "New Item Data"=w336) -> (w334:T1)
        }
      }
      frame "Data: Change Controls" {
        n153 = Unbundle By Name(w340) -> ("FP.Controls"=w339:string[][], "FP.Selected VI Data"=w338:i32)
        n154 = in-place "In Place Element Structure" {
          in-place-border: w339 -> [w345]
          in-place-border: w338 -> [w343]
          n155 = in-place-cluster #11(w340) -> ("New Item Data"=w346:refnum<class "Item.lvclass">[])
          n156 = call "Set Control Properties.vi"("VI Index"=w343, "Controls"=w345, "Item Data"=w346) -> ("Item Data out"=w344:refnum<class "Item.lvclass">[])  [unwired: 8 in]
          n157 = in-place-cluster #11("New Item Data"=w344) -> (w342:T1)
        }
      }
      frame "Data: Add Copyright" {
        n158 = Unbundle By Name(w356) -> ("FP.Selected VI Data"=w350:i32, "Config.Copyright Delimiter"=w347:string, "Config.Copyright Path"=w355:path)
        n159 = Read from Text File(file (use dialog)=w355, error in=w358) -> (refnum out=w359:refnum<file>, text=w354:string, error out=w360:errorcluster)  [unwired: 2 in, 1 out]
        n160 = Equal?(x=w353, y="All") -> (x = y?=w351:bool)
        n161 = Close File(refnum=w359, error in=w360) -> (error out=w357:errorcluster)  [unwired: 1 out]
        n162 = Select(t=-1, s=w351, f=w350) -> (s? t:f=w348:i32)
        n163 = in-place "In Place Element Structure" {
          in-place-border: w357 -> [w368]
          in-place-border: [w367] -> w362
          in-place-border: w348 -> [w365]
          in-place-border: w354 -> [w364]
          in-place-border: w347 -> [w363]
          n164 = in-place-cluster #12(w356) -> ("New Item Data"=w369:refnum<class "Item.lvclass">[])
          n165 = call "Add Copyright.vi"("VI Index"=w365, "error in (no error)"=w368, "Copyright Delimiter"=w363, "Copyright Text"=w364, "Item Data"=w369) -> ("error out"=w367:errorcluster, "Item Data out"=w366:refnum<class "Item.lvclass">[])  [unwired: 5 in]
          n166 = in-place-cluster #12("New Item Data"=w366) -> (w361:T1)
        }
      }
      frame "Data: Cleanup" {
        # "Cleanup any data and references, here.\n(this is called automatically, by the Macro: Exit)"
        n167 = Unbundle By Name(w370) -> ("Core.Current VI Reference"=w371:refnum<vi>)
        n168 = Close Reference(reference=w371, error in (no error)=w373) -> (error out=w372:errorcluster)
      }
      frame "---------- UI ----------" {
        # "Do not put any code in this frame.\n(It is a separator no-op. You can make a copy of this frame to create a new UI frame)"
      }
      frame "UI: Initialize" {
        # "Initialize the User Interface, here.\n(this is called automatically, by the Macro: Init)"
        n169 = Unbundle By Name(w377) -> ("FP Refs.Controls"=w376:refnum<vi>)
        n170 = call "Set Table Colors.vi"("Controls Table Ref"=w376) -> ()  [unwired: 10 in, 1 out]
      }
      frame "UI: Uninitialize" {
        # "Uninitialize the User Interface, here.\n(this is called automatically, by the Macro: Exit)"
        n171 = Unbundle By Name(w388) -> ("FP Refs.Controls"=w387:refnum<vi>, "FP Refs.VI Tree"=w379:refnum<vi>)
        n172 = invoke on="Invoke Node" class="VI" method="Default Vals.Reinit All"(error in=w383) -> (error out=w384:errorcluster)  [unwired: 2 in, 2 out]
        n173 = invoke on="Invoke Node" class="Tree (strict)" method="Edit Tree Items.Delete"(reference=w379, error in=w384, "Delete Children"=TRUE ("Delete Children?")) -> (error out=w381:errorcluster)  [unwired: 2 in, 4 out]
        n174 = call "Format Header Columns.vi"("error in (no error)"=w381, "Sort Order"=0, "Sort Column"=-1, "Controls Table Ref"=w387) -> ("error out"=w380:errorcluster)  [unwired: 7 in]
      }
      frame "UI: Initialize Menu" {
        n175 = Unbundle By Name(w390) -> ("Config"=w389:T4)
        n176 = Current VI's Menubar() -> (w391:refnum<k9>)
        n177 = call "Initialize Menu Items.vi"("error in (no error)"=w393, "Config"=w389, "Menu Ref"=w391) -> ("error out"=w392:errorcluster)  [unwired: 8 in]
      }
      frame "UI: Menu Selection" {
        n178 = Current VI's Menubar() -> (w395:refnum<k9>)
        n179 = call "Process Menu Selection.vi"("error in (no error)"=w398, "Argument"=w394, "Menu Ref"=w395) -> ("error out"=w397:errorcluster, "State(s) to Enqueue"=w396:string)  [unwired: 7 in]
        n180 = call "Enqueue Multiple States.vi"("queue in"=w399, "State(s) at Back"=w396) -> ()  [unwired: 13 in, 1 out]
      }
      frame "UI: Cursor Set" {
        # "Argument"
        # "Set and Unset Cursor Busy.\n(Usage: \"UI: Cursor Set >> Busy|Idle\")"
        n181 = case shown="\"Idle\", Default" w401 {
          tunnel: w404 -> [w406 w408]
          tunnel: [w405 w407] -> w403
          frame "Idle", Default {
            n182 = call <vilib>:"Unset Busy.vi"("error in (no error)"=w406) -> ("error out"=w405:errorcluster)  [unwired: 10 in]
          }
          frame "Busy" {
            n183 = call <vilib>:"Set Busy.vi"("error in (no error)"=w408) -> ("error out"=w407:errorcluster)  [unwired: 9 in, 1 out]
          }
        }
      }
      frame "UI: Front Panel State" {
        # "Argument"
        # "Set Front Panel Open or Closed\n(Usage: \"UI: Front Panel State >> Open|Close\")"
        n184 = Unbundle By Name(w411) -> ("Core.Current VI Reference"=w410:refnum<vi>)
        n185 = case shown="\"Open\", \"Standard\", Default" w409 {
          tunnel: w413 -> [w420 w434 w446 w459 w472]
          tunnel: [w421 w435 w447 w460 w473] -> w412
          tunnel: w410 -> [w418 w432 w444 w457 w470]
          frame "Open", "Standard", Default {
            w414 = T14."Standard" ("State")
            n186 = property on="Property Node" class="VI"(reference=w418, error in=w420) -> (reference out=w417:refnum<vi>, error out=w419:errorcluster, "FP.State"=w416:T14)
            n187 = Not Equal?(x=w416, y=w414) -> (x != y?=w415:bool)
            n188 = case shown="False" w415 {
              tunnel: [w426 w427] -> w421
              tunnel: w419 -> [w425 w427]
              tunnel: w417 -> [w423 _]
              tunnel: w414 -> [w422 _]
              frame True {
                n189 = invoke on="Invoke Node" class="VI" method="FP.Open"(reference=w423, error in=w425, "Activate"=TRUE, "State"=w422) -> (error out=w426:errorcluster)  [unwired: 1 in, 4 out]
              }
              frame False {
              }
            }
          }
          frame "Close", "Closed" {
            n190 = property on="Property Node" class="VI"(reference=w432, error in=w434) -> (reference out=w431:refnum<vi>, error out=w433:errorcluster, "FP.State"=w429:T14)
            n191 = Not Equal?(x=w429, y=T14."Closed" ("Front Panel Window:State")) -> (x != y?=w428:bool)
            n192 = case shown="True" w428 {
              tunnel: [w436 w439] -> w435
              tunnel: w433 -> [w436 w438]
              tunnel: w431 -> [_ w437]
              frame False {
              }
              frame True {
                n193 = invoke on="Invoke Node" class="VI" method="FP.Close"(reference=w437, error in=w438) -> (error out=w439:errorcluster)  [unwired: 1 in, 2 out]
              }
            }
          }
          frame "Hidden", "Hide" {
            w440 = T14."Hidden" ("State")
            n194 = property on="Property Node" class="VI"(reference=w444, error in=w446) -> (reference out=w443:refnum<vi>, error out=w445:errorcluster, "FP.State"=w442:T14)
            n195 = Not Equal?(x=w442, y=w440) -> (x != y?=w441:bool)
            n196 = case shown="True" w441 {
              tunnel: [w451 w452] -> w447
              tunnel: w445 -> [w450 w452]
              tunnel: w443 -> [w449 _]
              tunnel: w440 -> [w448 _]
              frame True {
                n197 = invoke on="Invoke Node" class="VI" method="FP.Open"(reference=w449, error in=w450, "State"=w448) -> (error out=w451:errorcluster)  [unwired: 2 in, 4 out]
              }
              frame False {
              }
            }
          }
          frame "Minimize", "Minimized" {
            w453 = T14."Minimized" ("State")
            n198 = property on="Property Node" class="VI"(reference=w457, error in=w459) -> (reference out=w456:refnum<vi>, error out=w458:errorcluster, "FP.State"=w455:T14)
            n199 = Not Equal?(x=w455, y=w453) -> (x != y?=w454:bool)
            n200 = case shown="True" w454 {
              tunnel: [w464 w465] -> w460
              tunnel: w458 -> [w463 w465]
              tunnel: w456 -> [w462 _]
              tunnel: w453 -> [w461 _]
              frame True {
                n201 = invoke on="Invoke Node" class="VI" method="FP.Open"(reference=w462, error in=w463, "State"=w461) -> (error out=w464:errorcluster)  [unwired: 2 in, 4 out]
              }
              frame False {
              }
            }
          }
          frame "Maximize", "Maximized" {
            w466 = T14."Maximized" ("State")
            n202 = property on="Property Node" class="VI"(reference=w470, error in=w472) -> (reference out=w469:refnum<vi>, error out=w471:errorcluster, "FP.State"=w468:T14)
            n203 = Not Equal?(x=w468, y=w466) -> (x != y?=w467:bool)
            n204 = case shown="True" w467 {
              tunnel: [w477 w478] -> w473
              tunnel: w471 -> [w476 w478]
              tunnel: w469 -> [w475 _]
              tunnel: w466 -> [w474 _]
              frame True {
                n205 = invoke on="Invoke Node" class="VI" method="FP.Open"(reference=w475, error in=w476, "State"=w474) -> (error out=w477:errorcluster)  [unwired: 2 in, 4 out]
              }
              frame False {
              }
            }
          }
        }
      }
      frame "UI: Panel Updates" {
        n206 = Unbundle By Name(w486) -> ("Core.Current VI Reference"=w485:refnum<vi>)
        n207 = Equal?(x=w481, y="Defer") -> (x = y?=w479:bool)
        n208 = property on="Property Node" class="VI"(reference=w485, error in=w483) -> (error out=w487:errorcluster, "Panel"=w484:refnum<vi>)  [unwired: 1 out]
        n209 = property on="Property Node" class="Pnl"(reference=w484, error in=w487, "Defer Panel Updates"=w479) -> (error out=w482:errorcluster)  [unwired: 1 out]
      }
      frame "UI: Interlocks" {
        n210 = Unbundle By Name(w494) -> ("FP Refs"=w488:T2, "New Item Data"=w493:refnum<class "Item.lvclass">[], "FP.Selected VI Data"=w490:i32)
        n211 = Current VI's Menubar() -> (w489:refnum<k9>)
        n212 = call "UI Interlocks.vi"("FP Refs"=w488, "error in (no error)"=w492, "Menu Ref"=w489, "VI Selected"=w490, "New Item Data"=w493) -> ("error out"=w491:errorcluster)  [unwired: 6 in]
      }
      frame "UI: Dialog" {
        n213 = call "Display Dialog.vi"("error in (no error)"=w501, "Argument"=w497, "State Data"=w499) -> ("error out"=w500:errorcluster, "States at Back"=w496:string, "States at Front"=w495:string, "State Data out"=w498:T1)  [unwired: 5 in]
        n214 = call "Enqueue Multiple States.vi"("State(s) at Front"=w495, "queue in"=w502, "State(s) at Back"=w496) -> ()  [unwired: 12 in, 1 out]
      }
      frame "UI: Format Item Names" {
        n215 = Unbundle By Name(w523) -> ("Displayed Indices"=w505:i32[], "Config.Abbreviate Names?"=w507:bool, "Config.Flat View?"=w506:bool, "New Item Data"=w511:refnum<class "Item.lvclass">[], "Saved Item Data"=w510:refnum<class "Item.lvclass">[], "FP Refs.VI Tree"=w513:refnum<vi>)
        n216 = call "Check Items for Modifications.vi"("Saved Item Data"=w510, "New Item Data"=w511) -> ("Number of Modified Items"=w508:i32, "New Item Data w/ Mod Bit Set"=w509:refnum<class "Item.lvclass">[])  [unwired: 8 in]
        n217 = call "Init Tree.vi"("error in"=w514) -> ("error out"=w516:errorcluster, "Tree Map out"=w517:refnum<class "Project Tree Map.lvclass">)  [unwired: 9 in]
        n218 = call "Format Item Names.vi"("Displayed Indices"=w505, "Flat View?"=w506, "Abbreviate Names?"=w507, "New Item Data"=w509) -> ("Number of Items Added"=w503:i32, "Formatted VI Data to Display"=w504:refnum<class "Item.lvclass">[])  [unwired: 6 in]
        n219 = call "Add Entries.vi"("error in"=w516, "Item Data"=w504, "Tree Map in"=w517) -> ("error out"=w515:errorcluster, "Tree Map out"=w512:refnum<class "Project Tree Map.lvclass">)  [unwired: 7 in]
        n220 = call "Build Tree.vi"("Tree"=w513, "error in"=w515, "Tree Map in"=w512) -> ("error out"=w518:errorcluster)  [unwired: 7 in, 1 out]
        n221 = call "Convert Item Count to Number String.vi"("Item Count"=w503) -> ("Number of Items String"=w520:string)  [unwired: 10 in]
        n222 = call "Convert Item Count to Number String.vi"("Item Count"=w508) -> ("Number of Items String"=w519:string)  [unwired: 10 in]
        n223 = Format Into String(format string="%s shown  -  %s modified", w520, w519) -> (resulting string=→"Current Counts":string)  [unwired: 2 in, 1 out]
      }
      frame "UI: Display Data" {
        n224 = Unbundle By Name(w529) -> ("Selected Item"=w524:refnum<class "Item.lvclass">, "FP Refs"=w525:T2, "Config"=w526:T4)
        n225 = call-dynamic "Display Item Info.vi"("error in (no error)"=w528, "Config"=w526, "Control References"=w525, "Item in"=w524) -> ("error out"=w527:errorcluster)  [unwired: 6 in, 1 out]
      }
      frame "UI: Select Source" {
        # "catch cancel error"
        n226 = case shown="\"File\"" w531 {
          tunnel: [_ w548 w554] -> w543
          tunnel: [_ w547 w553] -> w540
          tunnel: [TRUE ("cancelled") w546 w552] -> w539
          frame Default {
          }
          frame "Folder" {
            n227 = call "File Dialog"("prompt"="Select the directory of VIs to update") -> ("selected path"=w547:path, "cancelled"=w546:bool, "error out"=w548:errorcluster)  [unwired: 11 in, 1 out]
          }
          frame "File" {
            n228 = call "File Dialog2"("prompt"="Select the project, library, or class VIs to update", "pattern (all files)"="*.lvproj;*.lvlib;*.lvclass", "pattern label"="Project, Library, or Class") -> ("selected path"=w553:path, "cancelled"=w552:bool, "error out"=w554:errorcluster)  [unwired: 9 in, 1 out]
          }
        }
        n229 = Format Into String(format string="UI: Cursor Set >> Busy\nData: Load VIs\nData: Update >> Reset VI Tree\nData: Update >> %s Config\nData: Write Config\nUI: Initialize Menu\nData: Filter/Sort VIs\nMacro: Load VI\nUI: Format Item Names\nUI: Cursor Set >> Idle", w531) -> (resulting string=w530:string)  [unwired: 2 in, 1 out]
        n230 = Select(t="" ("Empty String Constant"), s=w539, f=w530) -> (s? t:f=w537:string)
        n231 = call <vilib>:"Clear Errors.vi"("error in (no error)"=w543, "specific error code to clear (0: all)"=43) -> ("error out"=w534:errorcluster)  [unwired: 4 in, 1 out]
        n232 = call "Enqueue Multiple States.vi"("queue in"=w544, "State(s) at Back"=w537) -> ()  [unwired: 13 in, 1 out]
        n233 = Merge Errors(w535, w534) -> (w533:errorcluster)
        n234 = Bundle By Name(cluster=w542, "Current Path"=w540) -> (w541:T1)
      }
      frame "UI: Open VI" {
        n235 = Unbundle By Name(w560) -> ("New Item Data"=w559:refnum<class "Item.lvclass">[], "FP.Selected VI Data"=w558:i32)
        n236 = Index Array(array=w559, index=w558) -> (element=w557:refnum<class "Item.lvclass">)
        n237 = property on="Property Node" class="Item.lvclass"(reference=w557) -> ("Accessors:Path"=w556:path)  [unwired: 1 in, 2 out]
        n238 = case shown="0, Default" w558 {
          tunnel: w562 -> [w566 w571]
          tunnel: [w565 w571] -> w561
          tunnel: w556 -> [w564 _]
          frame 0, Default {
            # "0x01 Record modifications\n0x02 Open templates for editing\n0x04 Prompt user to save"
            # "Open selected VI"
            n239 = Open VI Reference(vi path=w564, options=7, error in (no error)=w566) -> (vi reference=w568:refnum<vi>, error out=w567:errorcluster)  [unwired: 3 in]
            n240 = invoke on="Invoke Node" class="VI" method="FP.Open"(reference=w568, error in=w567) -> (reference out=w570:refnum<vi>, error out=w569:errorcluster)  [unwired: 3 in, 3 out]
            n241 = Close Reference(reference=w570, error in (no error)=w569) -> (error out=w565:errorcluster)
          }
          frame -1 {
            # "No VI selected, so do nothing"
          }
        }
      }
      frame "UI: Edit Copyright" {
        n242 = Unbundle By Name(w573) -> ("Config.Copyright Path"=w572:path)
        n243 = Format Into String(format string="Notepad.exe %s", error in=w575, w572) -> (resulting string=w578:string, error out=w579:errorcluster)  [unwired: 1 in]
        n244 = call <vilib>:"System Exec.vi"("wait until completion? (T)"=FALSE, "error in (no error)"=w579, "command line"=w578) -> ("error out"=w574:errorcluster)  [unwired: 5 in, 3 out]
      }
      frame "UI: Add Bold Tags" {
        n245 = control-ref of="VI description"() -> (w589:refnum<vi>)
        n246 = property on="Property Node" class="Str"(reference=w589, error in=w581) -> (reference out=w586:refnum<vi>, error out=w590:errorcluster, "Value"=w588:string, "Text.Selection"=w587:T8)
        n247 = call "Add Bold Tags.vi"("Selection"=w587, "Value"=w588) -> ("Selection out"=w585:T8, "Value out"=w582:string)  [unwired: 8 in]
        n248 = property on="Property Node" class="Str"(reference=w586, error in=w590, "Value"=w582, "Text.Selection"=w585) -> (error out=w580:errorcluster)  [unwired: 1 out]
        n249 = Bundle By Name(cluster=w584, "FP.VI Desc"=w582) -> (w583:T1)
      }
      frame "UI: Remove Bold Tags" {
        n250 = control-ref of="VI description"() -> (w600:refnum<vi>)
        n251 = property on="Property Node" class="Str"(reference=w600, error in=w592) -> (reference out=w597:refnum<vi>, error out=w601:errorcluster, "Value"=w599:string, "Text.Selection"=w598:T8)
        n252 = call "Remove Bold Tags.vi"("Selection"=w598, "Value"=w599) -> ("Selection out"=w596:T8, "Value out"=w593:string)  [unwired: 8 in]
        n253 = property on="Property Node" class="Str"(reference=w597, error in=w601, "Value"=w593, "Text.Selection"=w596) -> (error out=w591:errorcluster)  [unwired: 1 out]
        n254 = Bundle By Name(cluster=w595, "FP.VI Desc"=w593) -> (w594:T1)
      }
      frame "UI: Focus Desc" {
        n255 = control-ref of="VI description"() -> (w606:refnum<vi>)
        n256 = property on="Property Node" class="Str"(reference=w606, error in=w607, "Key Focus"=TRUE, "Text.Selection Start"=u32 4294967295 ("Text.Selection:End")) -> (error out=w602:errorcluster)  [unwired: 1 out]
      }
      frame "UI: Format Desc" {
        n257 = control-ref of="VI description"() -> (w613:refnum<vi>)
        n258 = Unbundle By Name(w610) -> ("Config.Format Bold Tags?"=w609:bool, "Desc Selection"=w608:T8)
        n259 = in-place "In Place Element Structure" {
          in-place-border: [w623] -> w615
          in-place-border: w614 -> [w622]
          in-place-border: w613 -> [w621]
          in-place-border: w612 -> [w620]
          in-place-border: w609 -> [w617]
          in-place-border: w608 -> [w616]
          n260 = in-place-cluster #13(w610) -> ("FP.VI Desc"=w619:string)
          n261 = case shown="\"Style\", Default" w620 {
            tunnel: [w624 w640] -> w623
            tunnel: w622 -> [w627 w639]
            tunnel: w621 -> [w626 w638]
            tunnel: w619 -> [_ w636]
            tunnel: [w633 w636] -> w618
            tunnel: w617 -> [w632 w637]
            tunnel: w616 -> [_ w635]
            frame "Tags" {
              n262 = call "Reset Plain Formatting.vi"("error in (no error)"=w627, "String Ref"=w626) -> ("error out"=w628:errorcluster, "String Ref out"=w625:refnum<vi>)  [unwired: 8 in]
              n263 = call "Find Bold Formatting.vi"("error in (no error)"=w628, "String Ref"=w625) -> ("error out"=w634:errorcluster, "Length"=w629:i32[], "Start"=w630:i32[], "String Ref out"=w631:refnum<vi>)  [unwired: 6 in]
              n264 = call "Replace Formatting with Tags.vi"("Set Value? (T)"=w632, "error in (no error)"=w634, "Length"=w629, "Start"=w630, "String Ref"=w631) -> ("error out"=w624:errorcluster, "New String"=w633:string)  [unwired: 4 in, 1 out]
            }
            frame "Style", Default {
              n265 = case shown="True" w637 {
                tunnel: [w641 w646] -> w640
                tunnel: w639 -> [w641 w645]
                tunnel: w638 -> [_ w644]
                tunnel: w636 -> [_ w643]
                tunnel: w635 -> [_ w642]
                frame False {
                }
                frame True {
                  n266 = call "Bold Description String.vi"("error in (no error)"=w645, "Selection"=w642, "String"=w643, "String Ref"=w644) -> ("error out"=w646:errorcluster)  [unwired: 7 in]
                }
              }
            }
          }
          n267 = in-place-cluster #13("FP.VI Desc"=w618) -> (w611:T1)
        }
      }
      frame "UI: Format Table Headers" {
        n268 = Unbundle By Name(w649) -> ("Config.Ctls Sort Column"=w648:i32, "Config.Ctls Sort Order"=w647:i32)
        n269 = in-place "In Place Element Structure" {
          in-place-border: [w657] -> w653
          in-place-border: w652 -> [w658]
          in-place-border: w651 -> [_]
          in-place-border: w648 -> [w655]
          in-place-border: w647 -> [w654]
          n270 = in-place-cluster #14(w649) -> ("FP Refs.Controls"=w656:refnum<vi>)
          n271 = call "Format Header Columns.vi"("error in (no error)"=w658, "Sort Order"=w654, "Sort Column"=w655, "Controls Table Ref"=w656) -> ("error out"=w657:errorcluster)  [unwired: 7 in]
          n272 = in-place-cluster #14("FP Refs.Controls"=w656) -> (w650:T1)
        }
      }
      frame "---------- Macro ----------" {
        # "Do not put any code in this frame.\n(It is a separator no-op. You can make a copy of this frame to create a new Macro frame)"
      }
      frame "Macro: Initialize" {
        w661 = "Data: Initialize\nInitialize Core Data\nData: Bundle Refs\nData: Read Config\nUI: Initialize\nUI: Format Table Headers\nUI: Interlocks\nUI: Front Panel State >> Open\nUI: Initialize Menu"  # Data: Initialize Initialize Core Data Data: Bundle Refs Data: Read Config UI: Initialize UI: Format Table Headers UI: Interlocks UI: Front Panel State >> Open UI: Initialize Menu
        # "Initialization Macro\n(This is called once, when the VI starts)"
        n273 = call "Enqueue Multiple States.vi"("State(s) at Front"=w661, "queue in"=w662) -> ()  [unwired: 13 in, 1 out]
      }
      frame "Macro: Load VI" {
        n274 = call "Enqueue Multiple States.vi"("State(s) at Front"="UI: Panel Updates >> Defer\nData: Update >> Selected Item\nData: Update >> All Ctls\nUI: Display Data\nUI: Format Desc\nUI: Panel Updates >> Undefer\nUI: Interlocks", "queue in"=w666) -> ()  [unwired: 13 in, 1 out]
      }
      frame "Macro: Load Recent Source" {
        n275 = case shown="\"Current\"" w670 {
          selector: w670 -> [_ w676]
          tunnel: ["UI: Cursor Set >> Busy\nData: Load VIs >> Reload\nUI: Initialize Menu\nData: Filter/Sort VIs\nMacro: Load VI\nUI: Format Item Names\nUI: Cursor Set >> Idle" w675] -> w669
          frame "Current" {
            # "Load source from Reload Source"
          }
          frame Default {
            # "Load source from Recent Files or Recent Folders"
            n276 = Search/Split String(string=w676, search string/char (-)="_") -> (substring before match=w678:string)  [unwired: 1 in, 2 out]
            n277 = Format Into String(format string="UI: Cursor Set >> Busy\nData: Update >> Reset VI Tree\nData: Update >> %s\nData: Update >> %s Config\nData: Load VIs\nData: Write Config\nUI: Initialize Menu\nData: Filter/Sort VIs\nMacro: Load VI\nUI: Format Item Names\nUI: Cursor Set >> Idle", w676, w678) -> (resulting string=w675:string)  [unwired: 2 in, 1 out]
          }
        }
        n278 = call "Enqueue Multiple States.vi"("State(s) at Front"=w669, "queue in"=w671) -> ()  [unwired: 13 in, 1 out]
      }
      frame "Macro: Revert" {
        n279 = case shown="\"\", Default" w682 {
          tunnel: ["Data: Revert Current\nUI: Format Item Names\nMacro: Load VI" "Data: Revert All\nUI: Format Item Names\nMacro: Load VI"] -> w683
          frame "", Default {
          }
          frame "All" {
          }
        }
        n280 = call "Enqueue Multiple States.vi"("State(s) at Front"=w683, "queue in"=w684) -> ()  [unwired: 13 in, 1 out]
      }
      frame "Macro: Save" {
        n281 = case shown="\"\", Default" w689 {
          tunnel: ["UI: Cursor Set >> Busy\nData: Save Current\nData: Update >> ItemsEdited\nData: Write Config\nUI: Format Item Names\nUI: Interlocks\nUI: Cursor Set >> Idle" "UI: Cursor Set >> Busy\nData: Save Current\nData: Update >> ItemsEdited\nData: Write Config\nUI: Format Item Names\nUI: Interlocks\nData: Update >> Inc Index\nMacro: Load VI\nUI: Cursor Set >> Idle\nUI: Focus Desc" "UI: Cursor Set >> Busy\nData: Save All\nData: Update >> ItemsEdited\nData: Write Config\nUI: Format Item Names\nUI: Interlocks\nUI: Cursor Set >> Idle" "UI: Cursor Set >> Busy\nData: Save All\nData: Update >> ItemsEdited\nData: Write Config\nUI: Format Item Names\nUI: Interlocks\nUI: Cursor Set >> Idle\nMacro: Exit"] -> w690
          frame "", Default {
          }
          frame "Go Next" {
          }
          frame "All" {
          }
          frame "Exit" {
          }
        }
        n282 = call "Enqueue Multiple States.vi"("State(s) at Front"=w690, "queue in"=w691) -> ()  [unwired: 13 in, 1 out]
      }
      frame "Macro: Exit" {
        # "Exit Macro\n(This is called once, when the VI exits)"
        n283 = Unbundle By Name(w707) -> ("Core.Close Panel on Exit?"=w706:bool)
        n284 = Generate User Event(user event=w699, event data cluster=FALSE ("event data"), error in=w708) -> (error out=w696:errorcluster)  [unwired: 1 in, 1 out]
        n285 = Select(t="UI: Front Panel State >> Close\n", s=w706, f="" ("Empty String Constant")) -> (s? t:f=w702:string)
        n286 = Concatenate Strings("UI: Uninitialize\n", w702, "Data: Cleanup\nExit") -> (w700:string)
        n287 = call "Enqueue Multiple States.vi"("State(s) at Front"=w700, "queue in"=w703) -> ()  [unwired: 13 in, 1 out]
      }
    }
  }
  n288 = Merge Errors(w9, w10) -> (w8:errorcluster)
  n289 = Release Queue(queue=w7, error in (no error)=w8) -> ()  [unwired: 1 in, 3 out]
